vi "motor_dc_registro_datos.vi"() -> ()   [LabVIEW 2010]
uses:
  <vilib>/DAQmx/read.llb/DAQmx Read (Counter U32 1Chan 1Samp).vi
  <vilib>/DAQmx/write.llb/DAQmx Write (Analog DBL 1Chan 1Samp).vi
  <vilib>/measure/madcrms.llb/Basic Averaged DC-RMS for 1 Chan.vi
  <vilib>/daqmx/miscellaneous.llb/DAQmx Fill In Error Info.vi
  <vilib>/measure/NI_MAPro.lvlib
panel:
  in  "File Name":path=path "C:/Documents and Settings/Administrador/Mis documentos/materiales cursos/Instrumentación/Material_clases/DAQ/data_motor_dc.lvm"
  out "XY Graph":cluster{"Y":dbl[], "Y":dbl[]}[](graph)=[{"Y"=[0.0, 0.5, 1.0, 1.5, 2.0, 2.5, 3.0, 3.5, 4.0, 4.5, 5.0, 5.5, 6.0, 6.5, 7.0, 7.5, 8.0, 8.5, 9.0, 9.5, 10.0, 10.5, 11.34375, 11.5, 12.0, 12.5, 13.0, 13.5, 14.0, 14.5, 15.0, 15.5, 16.0, 16.5, 17.0, 17.5, 18.0, 18.5, 19.0, 19.5, 20.0, 20.5, 21.0, 21.5, 22.0, 22.5, 23.0, 23.5, 24.0, 24.5, 25.0, 25.5, 26.0, 26.5, 27.0, 27.5, 28.0, 28.5, 29.0, 29.5, 30.0, 30.5, 31.0, 31.5, 32.0], "Y"=[0.0, 3.3333333333333335, 0.0, 0.0, 0.0, 0.0, 0.0, 0.0, 0.0, 0.0, 0.0, 1580.0, 1766.6666666666667, 1776.6666666666667, 1766.6666666666667, 1773.3333333333333, 1770.0, 1773.3333333333333, 1773.3333333333333, 1770.0, 1776.6666666666667, 713.3333333333334, 42.02020202020202, 0.0, 0.0, 0.0, 0.0, 0.0, 0.0, 0.0, 0.0, 1583.3333333333333, 1770.0, 1776.6666666666667, 1770.0, 1773.3333333333333, 1776.6666666666667, 1770.0, 1776.6666666666667, 1776.6666666666667, 1773.3333333333333, 713.3333333333334, 20.0, 0.0, 0.0, 0.0, 0.0, 0.0, 0.0, 0.0, 0.0, 1583.3333333333333, 1773.3333333333333, 1776.6666666666667, 1773.3333333333333, 1773.3333333333333, 1776.6666666666667, 1773.3333333333333, 1780.0, 1776.6666666666667, 1776.6666666666667, 713.3333333333334, 50.0, 33.333333333333336, 0.0]}, {"Y"=[0.0, 0.5, 1.0, 1.5, 2.0, 2.5, 3.0, 3.5, 4.0, 4.5, 5.0, 5.5, 6.0, 6.5, 7.0, 7.5, 8.0, 8.5, 9.0, 9.5, 10.0, 10.5, 11.34375, 11.5, 12.0, 12.5, 13.0, 13.5, 14.0, 14.5, 15.0, 15.5, 16.0, 16.5, 17.0, 17.5, 18.0, 18.5, 19.0, 19.5, 20.0, 20.5, 21.0, 21.5, 22.0, 22.5, 23.0, 23.5, 24.0, 24.5, 25.0, 25.5, 26.0, 26.5, 27.0, 27.5, 28.0, 28.5, 29.0, 29.5, 30.0, 30.5, 31.0, 31.5, 32.0], "Y"=[0.79, 0.79, 0.79, 0.79, 0.79, 0.79, 0.79, 0.79, 0.79, 0.79, 2.67, 2.67, 2.67, 2.67, 2.67, 2.67, 2.67, 2.67, 2.67, 2.67, 0.79, 0.79, 0.79, 0.79, 0.79, 0.79, 0.79, 0.79, 0.79, 0.79, 2.67, 2.67, 2.67, 2.67, 2.67, 2.67, 2.67, 2.67, 2.67, 2.67, 0.79, 0.79, 0.79, 0.79, 0.79, 0.79, 0.79, 0.79, 0.79, 0.79, 2.67, 2.67, 2.67, 2.67, 2.67, 2.67, 2.67, 2.67, 2.67, 2.67, 0.79, 0.79, 0.79, 0.79, 0.79]}]
  out "Time has Elapsed":bool
  in  "T_voltaje_control":dbl=10.0
  out "frecuencia [c/seg]":dbl
  out "tiempo [t]":dbl=32.0
  out "rpm":dbl(knob) scale=0.0..3000.0
  out "t_lazo [dt]":dbl=0.5
  in  "stop":bool
  out "v_control":dbl(knob) scale=0.0..5.0
  # "Muestreo"
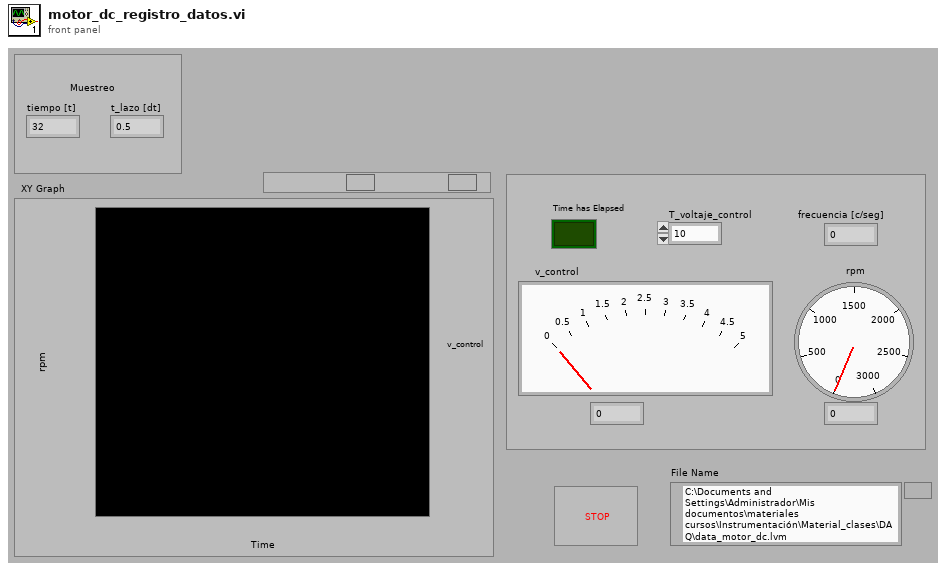
[diagram p1: front panel]
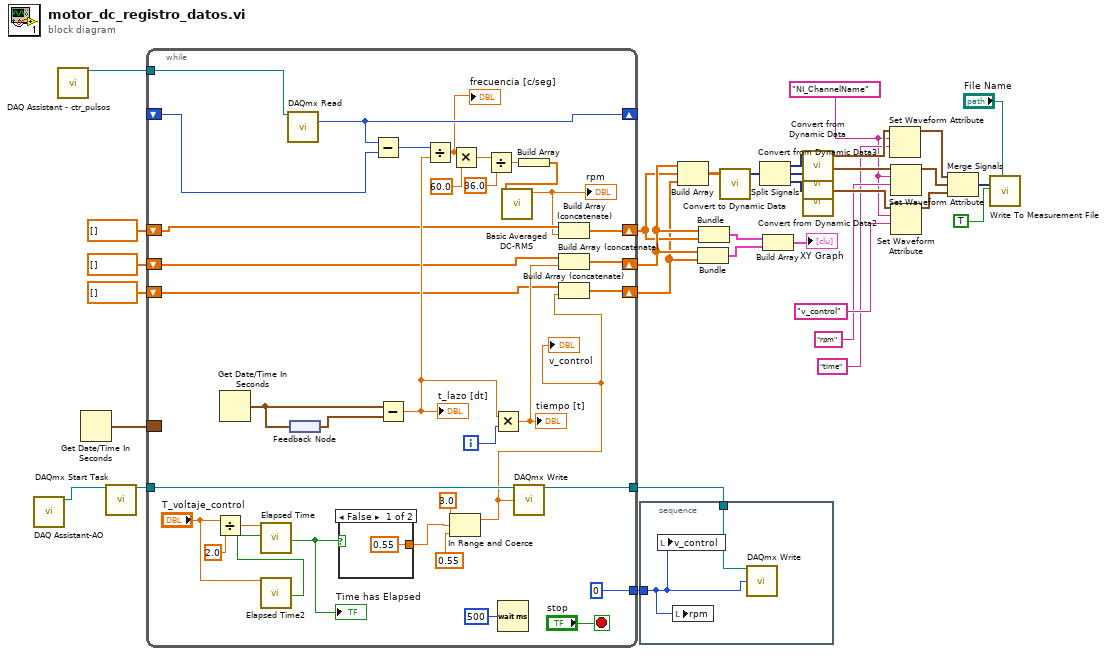
[diagram p0: block diagram]
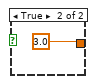
[diagram p2: hidden frame]
diagram:
  w1 = "NI_ChannelName" ("name")
  n1 = call "DAQ Assistant-AO"() -> ("task out"=w33:refnum<k21>)  [unwired: 4 in, 15 out]
  n2 = call "DAQ Assistant - ctr_pulsos"() -> ("task out"=w29:refnum<k21>)  [unwired: 3 in, 16 out]
  n3 = Get Date/Time In Seconds() -> (seconds since 1Jan1904=w28:timestamp)
  n4 = call <vilib>:"DAQmx Start Task.vi"("task/channels in"=w33) -> ("task out"=w32:refnum<k21>)  [unwired: 1 in, 13 out]
  n5 = while {
    tunnel: w32 -> [w68]
    tunnel: [0] -> w30
    tunnel: [w64] -> w31
    tunnel: w29 -> [w63]
    border: w28 -> [_]
    shift-right: [w59] -> _
    shift-left: _ -> [w58]
    shift-right: [w40] -> w20
    shift-left: dbl[] [] -> [w42]
    shift-right: [w37] -> w21
    shift-left: dbl[] [] -> [w38]
    shift-right: [w36] -> w18
    shift-left: dbl[] [] -> [w35]
    i -> [w50]
    stop <- "stop" stop-if-true
    n6 = Divide(x="T_voltaje_control", y=2.0) -> (x/y=w48:dbl)
    n7 = Get Date/Time In Seconds() -> (seconds since 1Jan1904=w61:timestamp)
    n8 = call "Elapsed Time2"("Time Target (s)"="T_voltaje_control") -> ("Time has Elapsed"=w45:bool)  [unwired: 4 in, 14 out]
    n9 = call "Elapsed Time"("Time Target (s)"=w48, "Reset"=w45) -> ("Time has Elapsed"=w44:bool)  [unwired: 3 in, 14 out]
    "Time has Elapsed" <- w44
    n10 = call-poly <vilib>:"DAQmx Read.vi"("task/channels in"=w63) -> ("data"=w59:u32)  [unwired: 1 in, 13 out]
    n11 = feedback-in #1(w61) -> ()
    n12 = feedback #1() -> (w60:timestamp)
    n13 = case shown="False" w44 {
      tunnel: [0.55 3.0] -> w43
      frame False {
      }
      frame True {
      }
    }
    n14 = Subtract(x=w59, y=w58) -> (x-y=w57:u32)
    n15 = Subtract(x=w61, y=w60) -> (x-y=w51:dbl)
    "t_lazo [dt]" <- w51
    n16 = Divide(x=w57, y=w51) -> (x/y=w49:dbl)
    "frecuencia [c/seg]" <- w49
    n17 = In Range and Coerce(upper limit=3.0, x=w43, lower limit=0.55) -> (coerced(x)=w34:dbl)  [unwired: 1 out]
    "v_control" <- w34
    n18 = Multiply(x=w49, y=60.0) -> (x*y=w55:dbl)
    n19 = Divide(x=w55, y=36.0) -> (x/y=w53:dbl)
    n20 = Multiply(x=w51, y=w50) -> (x*y=w39:dbl)
    "tiempo [t]" <- w39
    n21 = Wait (ms)(milliseconds to wait=u32 500) -> ()  [unwired: 1 out]
    n22 = call-poly <vilib>:"DAQmx Write.vi"("task/channels in"=w68, "data"=w34) -> ("task out"=w64:refnum<k21>)  [unwired: 2 in, 11 out]
    n23 = Build Array(w53) -> (w52:dbl[])
    n24 = call-poly <vilib>:"Basic Averaged DC-RMS.vi"("signal in"=w52) -> ("DC value"=w41:dbl)  [unwired: 5 in, 5 out]
    "rpm" <- w41
    n25 = Build Array (concatenate)(w42, w41) -> (w40:dbl[])
    n26 = Build Array (concatenate)(w38, w39) -> (w37:dbl[])
    n27 = Build Array (concatenate)(w35, w34) -> (w36:dbl[])
  }
  n28 = stacked-sequence {
    tunnel: w31 -> [w73]
    tunnel: w30 -> [w72]
    frame #0 {
      n29 = local write "v_control"(w72) -> ()
      n30 = local write "rpm"(w72) -> ()
      n31 = call-poly <vilib>:"DAQmx Write.vi"("task/channels in"=w73, "data"=w72) -> ()  [unwired: 2 in, 12 out]
    }
  }
  n32 = Build Array(w21, w20, w18) -> (w15:dbl[][])
  n33 = Bundle(w21, w18) -> (w23:cluster{dbl[], dbl[]})  [unwired: 1 out]
  n34 = Bundle(w21, w20) -> (w24:cluster{dbl[], dbl[]})  [unwired: 1 out]
  n35 = call "Convert to Dynamic Data"("2D Array"=w15) -> ("Dynamic Data Type"=w19:dynamicdata)  [unwired: 3 out]
  n36 = Split Signals(w19) -> (w14:dynamicdata, w13:dynamicdata, w12:dynamicdata)  [unwired: 3 out]
  n37 = Build Array(w24, w23) -> (→"XY Graph":cluster{dbl[], dbl[]}[])
  n38 = call "Convert from Dynamic Data"("Dynamic Data Type"=w14) -> ("Waveform"=w11:waveform(dbl))  [unwired: 1 in, 2 out]
  n39 = call "Convert from Dynamic Data3"("Dynamic Data Type"=w13) -> ("Waveform"=w10:waveform(dbl))  [unwired: 1 in, 2 out]
  n40 = call "Convert from Dynamic Data2"("Dynamic Data Type"=w12) -> ("Waveform"=w9:waveform(dbl))  [unwired: 1 in, 2 out]
  n41 = Set Waveform Attribute(5:"time", 6:w1, 7:w11) -> (3:w5:waveform(dbl))  [unwired: 1 in, 2 out]
  n42 = Set Waveform Attribute(5:"rpm", 6:w1, 7:w10) -> (3:w4:waveform(dbl))  [unwired: 1 in, 2 out]
  n43 = Set Waveform Attribute(5:"v_control", 6:w1, 7:w9) -> (3:w3:waveform(dbl))  [unwired: 1 in, 2 out]
  n44 = Merge Signals(w5, w4, w3) -> (w2:dynamicdata)
  n45 = call "Write To Measurement File"("Signals"=w2, "Enable"=TRUE, "File Name"="File Name") -> ()  [unwired: 4 in, 13 out]
